vi "get_steepest_slope_subvi.vi"(0 "sampling info":cluster{"Fs":dbl, "#s":dbl}, 5 "output cluster":T1) -> (4 "X derivative":waveform(dbl)(graph)={"t0"=timestamp(3564145341.961695 s since 1904-01-01), "dt"=0.0001999999998228304, "Y"=array[1000 elements], "attributes"=variant("NI_ChannelName"=variant(string "PXI1Slot4/ai1"), "NI_UnitDescription"=variant(string "Volts"))}, 6 "X":waveform(dbl)(graph)={"t0"=timestamp(3564145341.961695 s since 1904-01-01), "dt"=0.0001999999998228304, "Y"=array[1000 elements], "attributes"=variant("NI_ChannelName"=variant(string "PXI1Slot4/ai1"), "NI_UnitDescription"=variant(string "Volts"))}, 8 "Y":waveform(dbl)(graph)={"t0"=timestamp(3564145341.961695 s since 1904-01-01), "dt"=0.0001999999998228304, "Y"=array[1000 elements], "attributes"=variant("NI_ChannelName"=variant(string "PXI1Slot4/ai1"), "NI_UnitDescription"=variant(string "Volts"))}, 10 "peaks match":bool, 15 "max peak height":dbl)   [LabVIEW 2015]
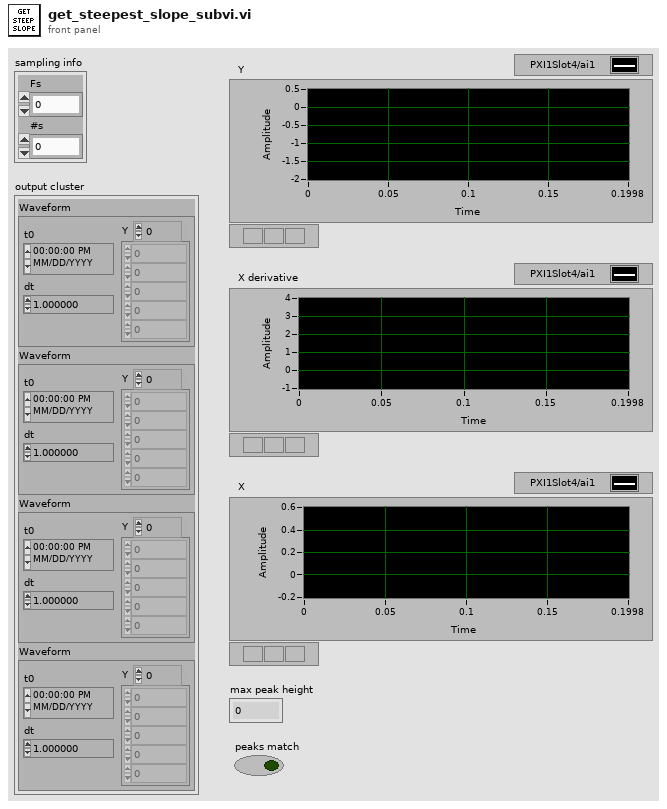
[diagram p1: front panel]
types:
  T1 = cluster{"Waveform":waveform(dbl), "Waveform":waveform(dbl), "Waveform":waveform(dbl), "Waveform":waveform(dbl)}
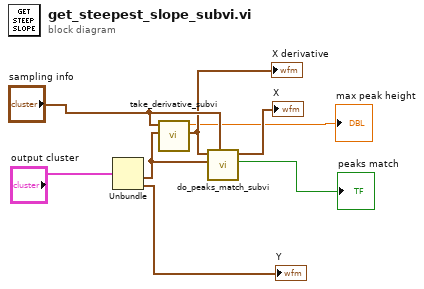
[diagram p0: block diagram]
diagram:
  n1 = Unbundle("output cluster") -> ("Waveform"=w5:waveform(dbl), "Waveform"=→"Y":waveform(dbl))  [unwired: 2 out]
  n2 = call "take_derivative_subvi.vi"("X in"=w5, "sampling info"="sampling info") -> ("derivative out"=w4:waveform(dbl), "max peak height"=→"max peak height":dbl)  [unwired: 8 in]
  "X derivative" <- w4
  n3 = call "do_peaks_match_subvi.vi"("derivative in"=w4, "X in"=w5, "sampling info"="sampling info") -> ("X out"=→"X":waveform(dbl), "peaks match"=→"peaks match":bool)  [unwired: 6 in]
